vi "valuePathv3.vi"(8 "error in (no error)":errorcluster, 9 "nodePath":string, 10 "value":string, 11 "xmlNode in":refnum<class "xmlNode.lvclass">) -> (0 "error out":errorcluster, 2 "Array":string[](array[string]), 3 "xmlNode out":refnum<class "xmlNode.lvclass">)   [LabVIEW 2009, in "Tools.lvlib" / "xml.lvlib" / "xmlNode.lvclass"]
doc: "Finds the xml struture leading to this value\ni.e. if I look for \"one\" I get /node1/node2/node3 from this example,\nand /node1/node4\n\n<node1>\n <node2>\n <node3>\"one\"</node3>\n </node2>\n <node4> \"one\" </node4>\n</node1>"
uses:
  xmlNode.lvclass
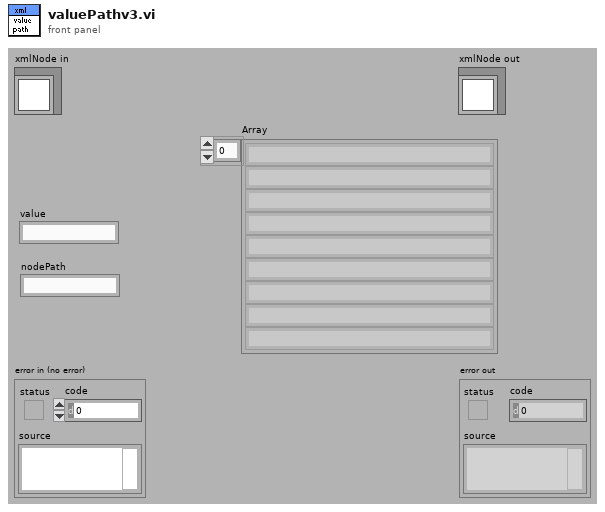
[diagram p1: front panel]
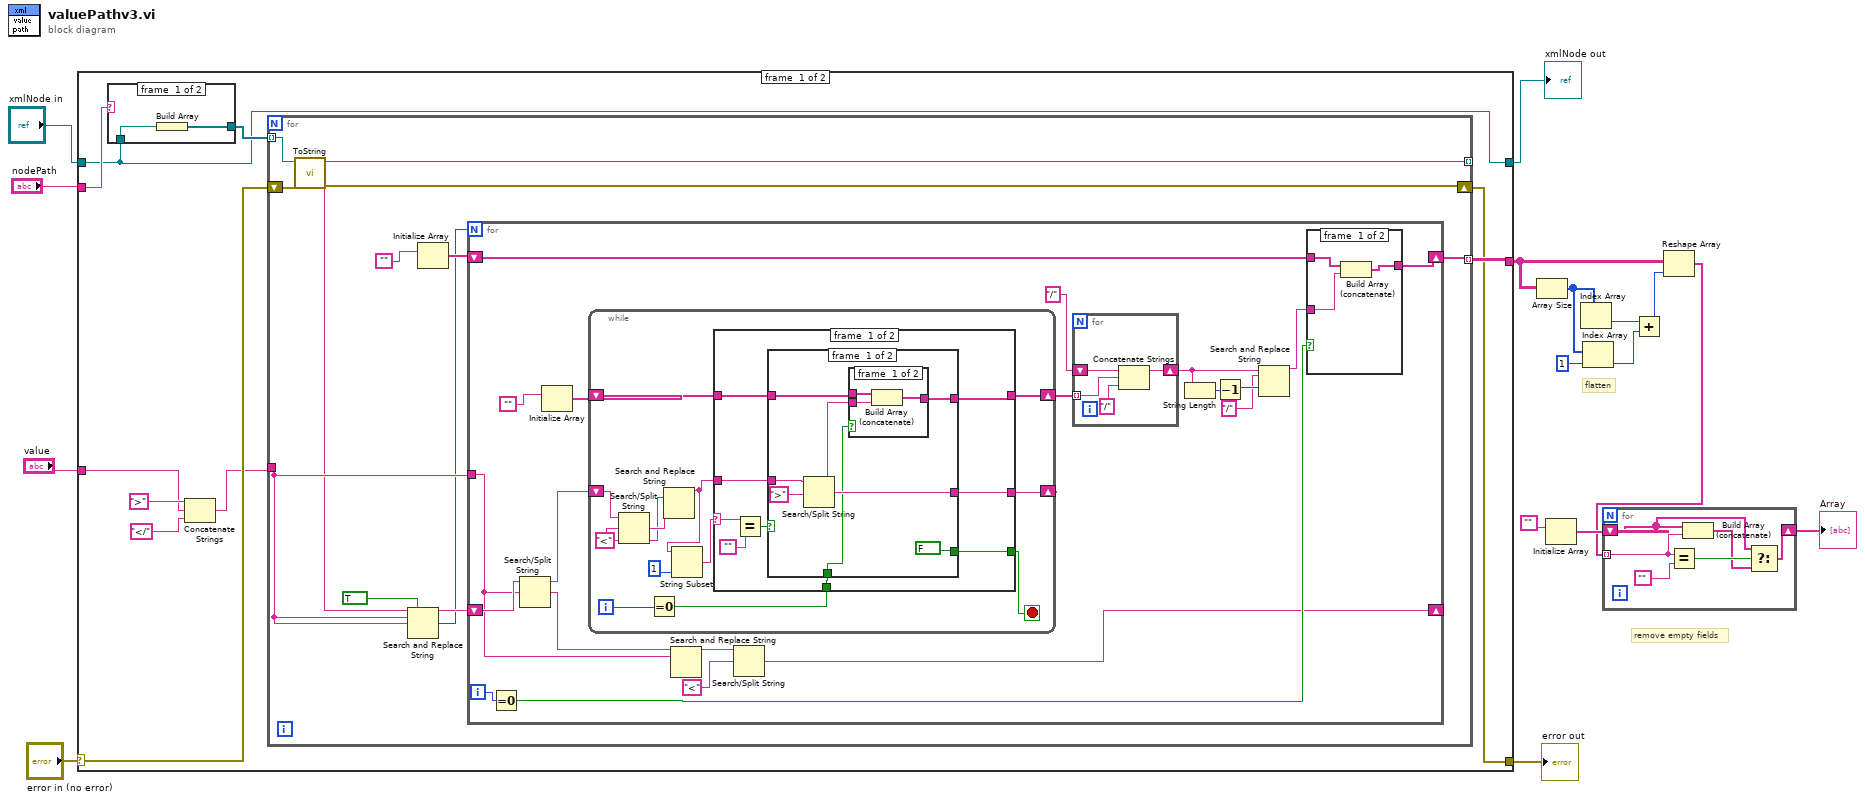
[diagram p0: block diagram]
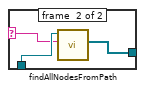
[diagram p2: hidden frame]
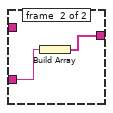
[diagram p3: hidden frame]
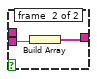
[diagram p4: hidden frame]
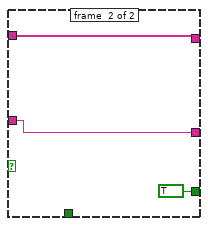
[diagram p5: hidden frame]
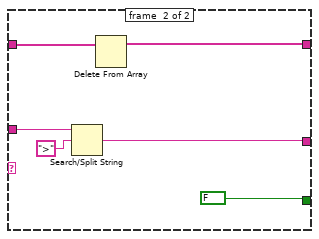
[diagram p6: hidden frame]
diagram:
  # "remove empty fields"
  # "flatten"
  n1 = case shown="No Error" "error in (no error)" {
    selector: "error in (no error)" -> [w21 w116]
    tunnel: [w24 w116] -> w16
    tunnel: [w22 w117] -> w15
    tunnel: "xmlNode in" -> [w22 w117]
    tunnel: [w26 _] -> w2
    tunnel: "value" -> [w18 _]
    tunnel: "nodePath" -> [w23 _]
    frame #0 {
      n2 = case shown="Default" w23 {
        selector: w23 -> [_ w29]
        tunnel: w22 -> [w28 w31]
        tunnel: [w27 w30] -> w25
        frame #0 {
          n3 = Build Array(w28) -> (w27:refnum<class "xmlNode.lvclass">[])
        }
        frame #1 {
          n4 = call "findAllNodesFromPath.vi"("nodePath"=w29, "xmlNode in"=w31) -> ("arrayXmlNodes"=w30:refnum<class "xmlNode.lvclass">[])  [unwired: 7 in, 2 out]
        }
      }
      n5 = Concatenate Strings(">", w18, "</") -> (w17:string)
      n6 = for {
        tunnel: [w43] -> w26 mode=indexing
        tunnel: w17 -> [w42]
        tunnel: [w41] -> _ mode=indexing
        tunnel: w25 -> [w39] mode=indexing
        shift-right: [w38] -> w24
        shift-left: w21 -> [w40]
        n7 = call-dynamic "ToString.vi"("error in (no error)"=w40, "xmlNode in"=w39) -> ("error out"=w38:errorcluster, "xml"=w35:string, "xmlNode out"=w41:refnum<class "xmlNode.lvclass">)  [unwired: 7 in]
        n8 = Search and Replace String(replace all?=TRUE, input string=w35, search string=w42, replace string=w42) -> (result string=w36:string, number of replacements=w32:i32)  [unwired: 4 in, 2 out]
        n9 = Initialize Array("") -> (w33:string[])  [unwired: 1 in]
        n10 = for {
          N: w32 -> [_]
          tunnel: w42 -> [w46]
          shift-right: [w44] -> _
          shift-left: w36 -> [w63]
          shift-right: [w57] -> w43
          shift-left: w33 -> [w56]
          i -> [w59]
          n11 = Equal To 0?(x=w59) -> (x = 0?=w58:bool)
          n12 = Search/Split String(string=w63, search string/char (-)=w46) -> (substring before match=w62:string, match + rest of string=w48:string)  [unwired: 1 in, 1 out]
          n13 = Initialize Array("") -> (w49:string[])  [unwired: 1 in]
          n14 = while {
            shift-right: [w78] -> w61
            shift-left: w49 -> [w79]
            shift-right: [w81] -> _
            shift-left: w62 -> [w84]
            i -> [w80]
            stop <- w76 stop-if-true
            w74 = "<"
            n15 = Search/Split String(string=w84, search string/char (-)=w74) -> (match + rest of string=w75:string)  [unwired: 1 in, 2 out]
            n16 = Equal To 0?(x=w80) -> (x = 0?=w77:bool)
            n17 = Search and Replace String(input string=w75, search string=w74) -> (result string=w73:string)  [unwired: 6 in, 3 out]
            n18 = String Subset(string=w73, length (rest)=1) -> (substring=w83:string)  [unwired: 1 in]
            n19 = case shown="Default" w83 {
              selector: w83 -> [w86 _]
              tunnel: w73 -> [w93 w114]
              tunnel: [w92 w112] -> w81
              tunnel: [w90 w111] -> w78
              tunnel: w79 -> [w91 w115]
              tunnel: w77 -> [w89 _]
              tunnel: [w88 FALSE] -> w76
              frame #0 {
                n20 = Equal?(x=w86, y="") -> (x = y?=w87:bool)
                n21 = case shown="False" w87 {
                  tunnel: w93 -> [w101 w108]
                  tunnel: [w99 w108] -> w92
                  tunnel: w91 -> [w98 w109]
                  tunnel: [w97 w109] -> w90
                  tunnel: w89 -> [w95 _]
                  tunnel: [FALSE TRUE] -> w88
                  frame #0 {
                    n22 = Search/Split String(string=w101, search string/char (-)=">") -> (substring before match=w96:string, match + rest of string=w99:string)  [unwired: 1 in, 1 out]
                    n23 = case shown="True" w95 {
                      tunnel: w96 -> [w103 w105]
                      tunnel: w98 -> [w102 _]
                      tunnel: [w104 w106] -> w97
                      frame #0 {
                        n24 = Build Array (concatenate)(w102, w103) -> (w104:string[])
                      }
                      frame #1 {
                        n25 = Build Array(w105) -> (w106:string[])
                      }
                    }
                  }
                  frame #1 {
                  }
                }
              }
              frame #1 {
                n26 = Search/Split String(string=w114, search string/char (-)=">") -> (match + rest of string=w112:string)  [unwired: 1 in, 2 out]
                n27 = Delete From Array(array=w115) -> (array with subset deleted=w111:string[])  [unwired: 2 in, 1 out]
              }
            }
          }
          n28 = Search and Replace String(input string=w48, search string=w46) -> (result string=w47:string)  [unwired: 6 in, 3 out]
          n29 = Search/Split String(string=w47, search string/char (-)="<") -> (match + rest of string=w44:string)  [unwired: 1 in, 2 out]
          n30 = for {
            tunnel: w61 -> [w71] mode=indexing
            shift-right: [w70] -> w52
            shift-left: "/" -> [w72]
            n31 = Concatenate Strings(w72, w71, "/") -> (w70:string)
          }
          n32 = String Length(string=w52) -> (length=w55:i32)
          n33 = Decrement(x=w55) -> (x-1=w54:i32)
          n34 = Search and Replace String(input string=w52, search string="/", offset=w54) -> (result string=w51:string)  [unwired: 5 in, 3 out]
          n35 = case shown="True" w58 {
            tunnel: w51 -> [w65 w68]
            tunnel: [w64 w67] -> w57
            tunnel: w56 -> [w66 _]
            frame #0 {
              n36 = Build Array (concatenate)(w66, w65) -> (w64:string[])
            }
            frame #1 {
              n37 = Build Array(w68) -> (w67:string[])
            }
          }
        }
      }
    }
    frame #1 {
    }
  }
  "error out" <- w16
  "xmlNode out" <- w15
  n38 = Array Size(array=w2) -> (size(s)=w10:i32[])
  n39 = Initialize Array("") -> (w4:string[])  [unwired: 1 in]
  n40 = Index Array(array=w10) -> (element=w8:i32)  [unwired: 1 in]
  n41 = Index Array(array=w10, index=1) -> (element=w7:i32)
  n42 = Add(x=w8, y=w7) -> (x+y=w6:i32)
  n43 = Reshape Array(w2, w6) -> (w3:string[])
  n44 = for {
    tunnel: w3 -> [w121] mode=indexing
    shift-right: [w118] -> w1
    shift-left: w4 -> [w119]
    n45 = Equal?(x=w121, y="") -> (x = y?=w122:bool)
    n46 = Build Array (concatenate)(w119, w121) -> (w120:string[])
    n47 = Select(t=w119, s=w122, f=w120) -> (s? t:f=w118:string[])
  }
  "Array" <- w1
